vi "get image handle.vi"(8 "error in (no error)":errorcluster, 11 "Cascade in":refnum<class "Cascade.lvclass">) -> (0 "error out":errorcluster, 3 "Cascade out":refnum<class "Cascade.lvclass">)   [LabVIEW 2012, in "Cascade.lvclass"]
uses:
  Cascade.lvclass
  Cascade.lvclass/Cascade.ctl
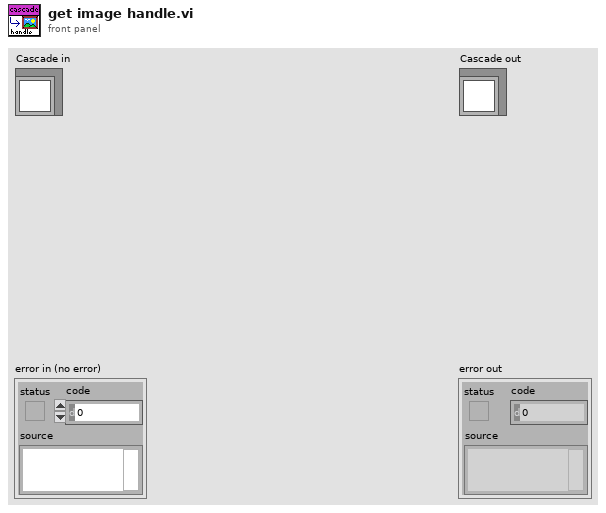
[diagram p1: front panel]
types:
  T1 = typedef "Cascade.lvclass/data type.ctl" = u32
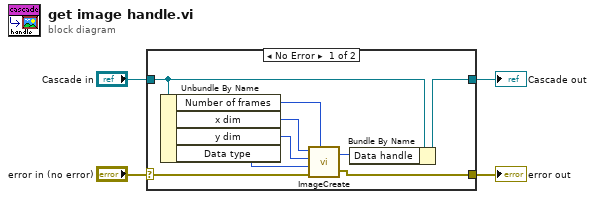
[diagram p0: block diagram]
diagram:
  n1 = case shown="No Error" "error in (no error)" {
    selector: "error in (no error)" -> [w13 w15]
    tunnel: [w12 w15] -> w3
    tunnel: [w6 w14] -> w1
    tunnel: "Cascade in" -> [w7 w14]
    frame No Error {
      n2 = Unbundle By Name(w7) -> ("Number of frames"=w8:u32, "x dim"=w9:u32, "y dim"=w10:u32, "Data type"=w11:T1)
      n3 = call <userlib>:"ImageCreate.vi"("X dimension"=w9, "Y dimension"=w10, "Data Type"=w11, "error in"=w13, "Number Of Frames"=w8) -> ("Image Handle"=w5:u32, "error out"=w12:errorcluster)
      n4 = Bundle By Name(cluster=w7, "Data handle"=w5) -> (w6:refnum<class "Cascade.lvclass">)
    }
    frame Error {
    }
  }
  "error out" <- w3
  "Cascade out" <- w1
